vi "PTSequencer.edit step.vi"(0 "i ref in":refnum<vi>, 2 "Step":T1, 3 "ms timeout (10000)":i32=10000, 4 "index":i32, 5 "error in (no error)":errorcluster) -> (14 "i ref out":refnum<vi>, 17 "timed out":bool, 19 "error out":errorcluster)   [LabVIEW 2014, in "PTSequencer.lvlib"]
uses:
  PTSequencer.lvlib
  PTSequencer.step.ctl
  CSCore/CSSystem/CoreDefs/CoreDefs.rawDataType.ctl
  PTSequencer.DIM service condition.ctl
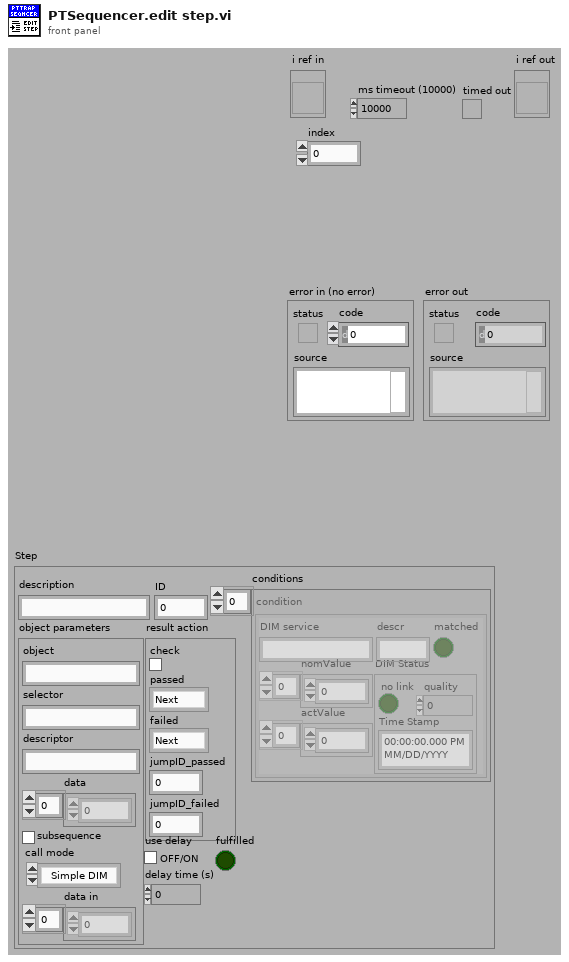
[diagram p1: front panel]
types:
  T1 = typedef "PTSequencer.lvlib/PTSequencer.step.ctl" = cluster{"description":string, "object parameters":cluster{"object":string, "selector":string, "descriptor":string, "data":T2, "subsequence":bool, "call mode":enum16{"Simple DIM", "Synchronous"}, "data in":T2}, "result action":cluster{"check":bool, "passed":enum16{"Next", "Previous", "Repeat", "Jump"}, "failed":enum16{"Next", "Previous", "Repeat", "Jump"}, "jumpID_passed":i32, "jumpID_failed":i32}, "conditions":T3[], "fulfilled ":bool, "use delay":bool, "delay time (s)":dbl, "ID":i32}
  T2 = typedef "CoreDefs.rawDataType.ctl" = i8[]
  T3 = typedef "PTSequencer.lvlib/PTSequencer.DIM service condition.ctl" = cluster{"DIM service":string, "descr":string, "nomValue":T2, "actValue":T2, "matched":bool, "DIM Status":cluster{"no link":bool, "quality":i32, "Time Stamp":timestamp}}
  T4 = typedef "PTSequencer.lvlib/PTSequencer.i attribute.ctl" = cluster{"subsequence":bool, "mode":T5, "i step":i32, "nofLoops":i32, "i loop":i32, "Running":bool, "Paused":bool, "step done":bool, "loop done":bool, "seq done":bool, "DIM IDs":cluster{"step done":i32, "loop done":i32, "seq done":i32, "i step":i32, "i loop":i32}, "use stop conditions":bool, "stop conditions":T3[], "Step List":T1[], "DIM subsriptions":string[], "stop cond indexes":i32[], "step cond indexes":cluster{"step condition IDs":cluster{"step ID":i32, "condition ID":i32}[]}[], "Delay Start Time":timestamp, "status":string, "stopping":bool}
  T5 = typedef "PTSequencer.lvlib/PTSequencer.mode.ctl" = enum16{"single", "loop", "for loop"}
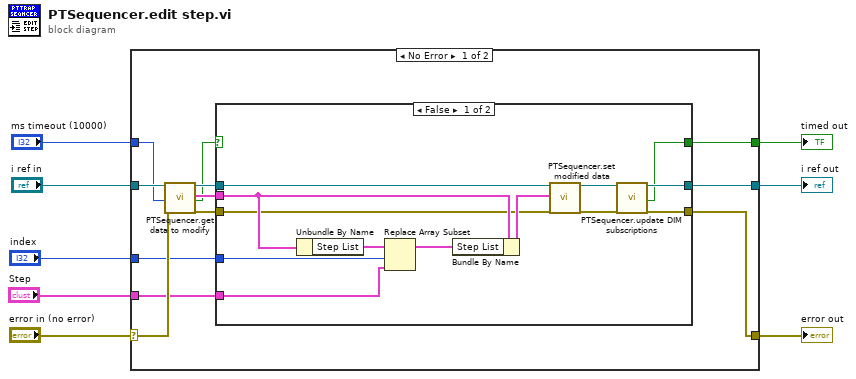
[diagram p0: block diagram]
diagram:
  n1 = case shown="No Error" "error in (no error)" {
    selector: "error in (no error)" -> [w15 w37]
    tunnel: "i ref in" -> [w20 w38]
    tunnel: [w10 w38] -> w7
    tunnel: [w11 w37] -> w5
    tunnel: "Step" -> [w14 _]
    tunnel: "index" -> [w13 _]
    tunnel: "ms timeout (10000)" -> [w12 _]
    tunnel: [w9 _] -> w1
    frame No Error {
      n2 = call "PTSequencer.get data to modify.vi"("i ref in"=w20, "ms timeout (10000)"=w12, "error in (no error)"=w15) -> ("i ref out"=w18:refnum<vi>, "i attribute"=w19:T4, "timed out"=w16:bool, "error out"=w17:errorcluster)  [unwired: 13 in]
      n3 = case shown="False" w16 {
        selector: w16 -> [_ w34]
        tunnel: w19 -> [w32 _]
        tunnel: w18 -> [w27 w36]
        tunnel: w17 -> [w26 w35]
        tunnel: [w22 w36] -> w10
        tunnel: [w23 w35] -> w11
        tunnel: w14 -> [w29 _]
        tunnel: w13 -> [w28 _]
        tunnel: [w21 w34] -> w9
        frame False {
          n4 = Unbundle By Name(w32) -> ("Step List"=w33:T1[])
          n5 = Replace Array Subset(array=w33, new element=w29, index=w28) -> (w31:T1[])
          n6 = Bundle By Name(cluster=w32, "Step List"=w31) -> (w30:T4)
          n7 = call "PTSequencer.set modified data.vi"("i ref in"=w27, "CLASS.i attribute"=w30, "error in (no error)"=w26) -> ("i ref out"=w25:refnum<vi>, "error out"=w24:errorcluster)  [unwired: 15 in]
          n8 = call "PTSequencer.update DIM subscriptions.vi"("i ref in"=w25, "error in"=w24) -> ("i ref out"=w22:refnum<vi>, "timed out"=w21:bool, "error out"=w23:errorcluster)  [unwired: 15 in]
        }
        frame True {
        }
      }
    }
    frame Error {
    }
  }
  "error out" <- w5
  "i ref out" <- w7
  "timed out" <- w1
